vi "develop run order.vi"(2 "error in (no error)":errorcluster, 3 "all rows":string[][](array[string]), 4 "number of samples between standards":i32=4) -> (0 "error out":errorcluster, 1 "Group run list":string[][](array[string]))   [LabVIEW 2016]
doc: "This is the main sub vi that sorts, arranges, and lists data in a run order"
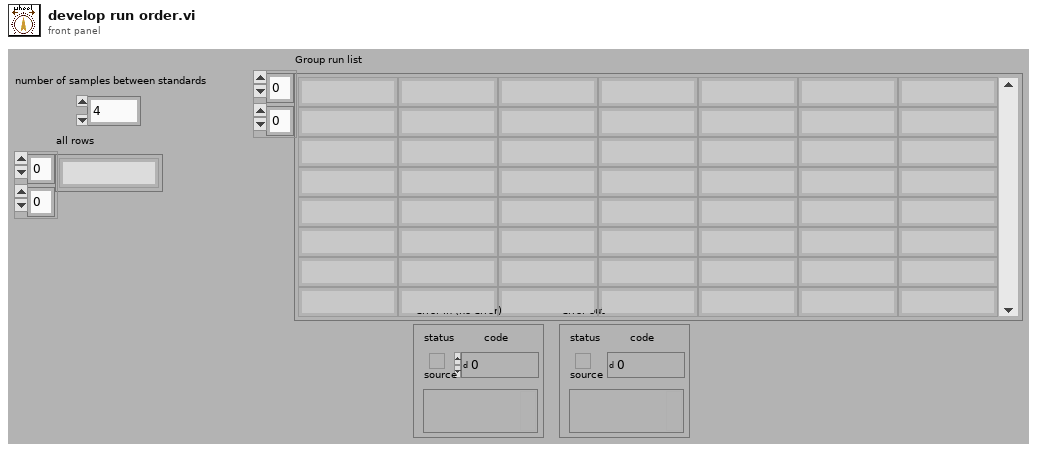
[diagram p1: front panel]
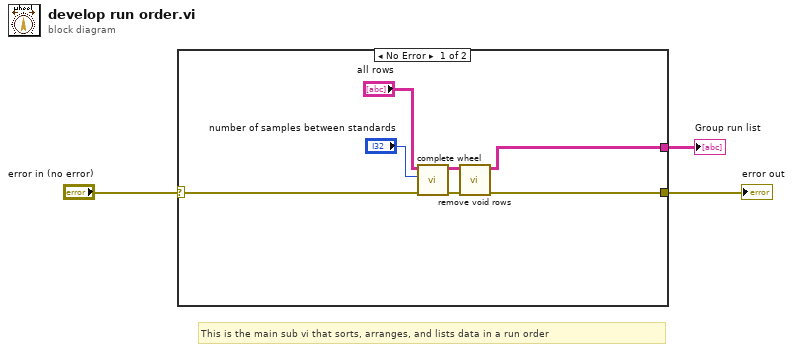
[diagram p0: block diagram]
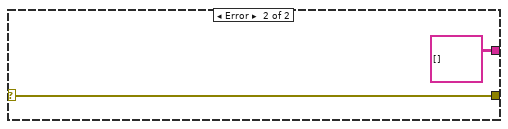
[diagram p2: hidden frame]
diagram:
  # "This is the main sub vi that sorts, arranges, and lists data in a run order"
  n1 = case shown="No Error" "error in (no error)" {
    selector: "error in (no error)" -> [w6 w11]
    tunnel: [w5 w11] -> w2
    tunnel: [w4 string[][] [] ("Group run list")] -> w1
    frame No Error {
      n2 = call "complete wheel.vi"("error in (no error)"=w6, "number of samples between standards"="number of samples between standards", "all rows"="all rows") -> ("error out"=w9:errorcluster, "Group run list"=w10:string[][])  [unwired: 7 in]
      n3 = call "remove void rows.vi"("error in"=w9, "Group run list input"=w10) -> ("error out"=w5:errorcluster, "Group run list"=w4:string[][])  [unwired: 8 in]
    }
    frame Error {
    }
  }
  "error out" <- w2
  "Group run list" <- w1
